vi "Processing_1DHistogram.vi"(4 "Minimum Log(G/G0) (-6)":dbl=-6.0, 5 "Reset":bool, 6 "Maximum Log(G/G0) (0.5)":dbl=0.5, 7 "Number of Bins (700)":i32=700, 8 "Error In":errorcluster, 10 "Enable?":bool, 11 "Log(G/G0)":dbl[](array[numeric])) -> (0 "Error Out":errorcluster, 1 "Enable? Out":bool, 3 "Histogram":i32[](array[numeric]))   [LabVIEW 2023]
panel:
  out "Waveform Graph":i32[](graph)
  in  "Array":i32[][](array[numeric])
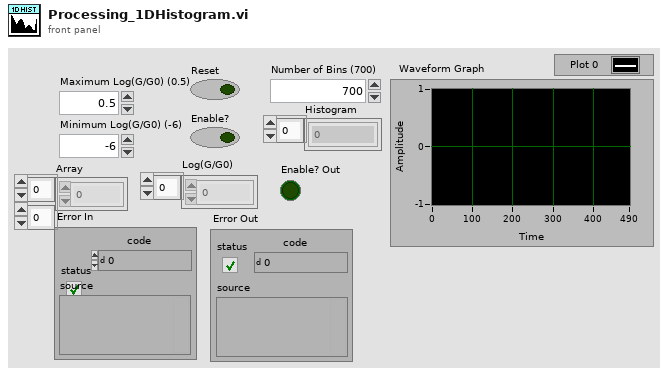
[diagram p1: front panel]
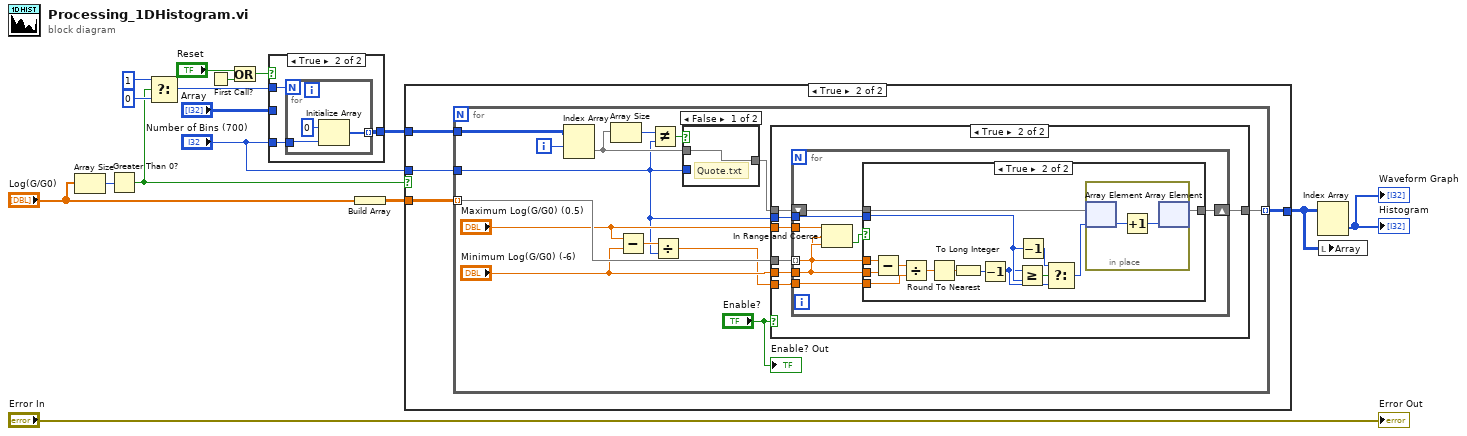
[diagram p0: block diagram]
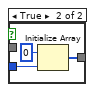
[diagram p5: hidden frame]
diagram:
  n1 = Array Size(array="Log(G/G0)") -> (size(s)=w2:i32)
  n2 = Greater Than 0?(x=w2) -> (x > 0?=w1:bool)
  n3 = Select(t=1, s=w1, f=0) -> (s? t:f=w3:i32)
  n4 = First Call?() -> (First Call?: T/F=w14:bool)
  n5 = Or(x="Reset", y=w14) -> (x .or. y?=w6:bool)
  n6 = case shown="True" w6 {
    tunnel: "Number of Bins (700)" -> [_ w20]
    tunnel: [w17 w19] -> w7
    tunnel: "Array" -> [w17 _]
    tunnel: w3 -> [_ w18]
    frame False {
      # "Cogito, ergo\nsum."
    }
    frame True {
      n7 = for {
        N: w18 -> [_]
        tunnel: w20 -> [w23]
        tunnel: [w22] -> w19 mode=indexing
        n8 = Initialize Array(0, w23) -> (w22:i32[])
      }
    }
  }
  n9 = Build Array("Log(G/G0)") -> (w10:dbl[][])
  n10 = case shown="True" w1 {
    tunnel: w7 -> [w24 w28]
    tunnel: w10 -> [_ w27]
    tunnel: [w24 w25] -> w9
    tunnel: "Number of Bins (700)" -> [_ w26]
    frame False {
      # "You, the legendary bravest of the brave, shall live out the rest of your days in abject fear,\nwatching helplessly as I bend the world to my will. Knowng you are utterly powerless to stop me,\nthat you are no longer important enough for me to destroy."
    }
    frame True {
      n11 = for {
        tunnel: w27 -> [w42] mode=indexing
        tunnel: w28 -> [w41]
        tunnel: w26 -> [w32]
        tunnel: [w31] -> w25 mode=indexing
        i -> [w30]
        n12 = Index Array(array=w41, index (row)=w30) -> (element=w38:i32[])  [unwired: 1 in]
        n13 = Array Size(array=w38) -> (size(s)=w40:i32)
        n14 = Subtract(x="Maximum Log(G/G0) (0.5)", y="Minimum Log(G/G0) (-6)") -> (x-y=w34:dbl)
        n15 = Not Equal?(x=w40, y=w32) -> (x != y?=w39:bool)
        n16 = Divide(x=w34, y=w32) -> (x/y=w33:dbl)
        n17 = case shown="False" w39 {
          tunnel: w32 -> [_ w78]
          tunnel: [w76 w77] -> w37
          tunnel: w38 -> [w76 _]
          frame False {
            # "Quote.txt"
          }
          frame True {
            n18 = Initialize Array(0, w78) -> (w77:i32[])
          }
        }
        n19 = case shown="True" "Enable?" {
          tunnel: "Minimum Log(G/G0) (-6)" -> [_ w50]
          tunnel: w42 -> [_ w49]
          tunnel: w37 -> [w43 w48]
          tunnel: [w43 w47] -> w31
          tunnel: "Maximum Log(G/G0) (0.5)" -> [_ w46]
          tunnel: w33 -> [_ w45]
          tunnel: w32 -> [_ w44]
          frame False {
            # "I've seen things you people wouldn't believe. \nAttack ships on fire off the shoulder of Orion.\nI watched C-beams glitter in the dark near the\n Tannhauser Gate. All those moments will be \nlost in time, like tears in rain."
          }
          frame True {
            n20 = for {
              tunnel: w49 -> [w53] mode=indexing
              tunnel: w50 -> [w54]
              tunnel: w45 -> [w58]
              shift-right: [w56] -> w47
              shift-left: w48 -> [w57]
              tunnel: w46 -> [w55]
              tunnel: w44 -> [w52]
              n21 = In Range and Coerce(upper limit=w55, x=w53, lower limit=w54) -> (In Range?=w51:bool)  [unwired: 1 out]
              n22 = case shown="True" w51 {
                tunnel: w58 -> [_ w72]
                tunnel: w57 -> [w59 w69]
                tunnel: [w59 w68] -> w56
                tunnel: w54 -> [_ w67]
                tunnel: w53 -> [_ w66]
                tunnel: w52 -> [_ w64]
                frame False {
                  # "I was never one to hold a grudge.\nMy Father held grudges, I'll always\nhate him for that."
                }
                frame True {
                  n23 = Subtract(x=w66, y=w67) -> (x-y=w73:dbl)
                  n24 = Divide(x=w73, y=w72) -> (x/y=w71:dbl)
                  n25 = Round To Nearest(number=w71) -> (nearest integer value=w70:dbl)
                  n26 = To Long Integer(number=w70) -> (32bit integer=w61:i32)
                  n27 = Decrement(x=w61) -> (x-1=w60:i32)
                  n28 = Greater Or Equal?(x=w60, y=w64) -> (x >= y?=w65:bool)
                  n29 = Decrement(x=w64) -> (x-1=w63:i32)
                  n30 = Select(t=w63, s=w65, f=w60) -> (s? t:f=w62:i32)
                  n31 = in-place {
                    n32 = in-place-array #1(w69, w62) -> (w74:i32)
                    n33 = Increment(x=w74) -> (x+1=w75:i32)
                    n34 = in-place-array #1(w75) -> (w68:i32[])  [unwired: 1 out]
                  }
                }
              }
            }
          }
        }
        "Enable? Out" <- "Enable?"
      }
    }
  }
  n35 = Index Array(array=w9) -> (element=→"Waveform Graph" →"Histogram":i32[])  [unwired: 2 in]
  n36 = local write "Array"(w9) -> ()
  "Error Out" <- "Error In"
